vi "FIR_4decimate_Filter2.vi"(8 "valid in":bool, 10 "Q in":fxp<+/-,16,14>, 11 "I in":fxp<+/-,16,14>) -> (0 "valid out":bool, 2 "Q out":fxp<+/-,16,14>, 3 "I out":fxp<+/-,16,14>)   [LabVIEW 2013]
uses:
  <vilib>/rvi/IPIntegrationNode/IPINode_Utilities/niFpgaIPINodeSimCore.vi
  <vilib>/rvi/XilinxIP/XIPIN_XNode/niFpgaXIPIN.xnode
  Filters/Polyphase filterbank/Filter2/Polyphase_filterbank_Filter2_155030D15C70440C8A7262E8A5168E06.dll
  <vilib>/rvi/IPIntegrationNode/IPINode_Xnode/niFpgaIPINode.xnode
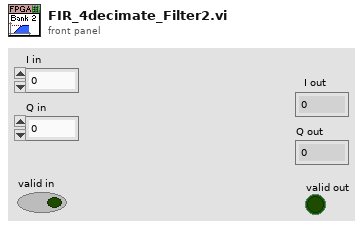
[diagram p1: front panel]
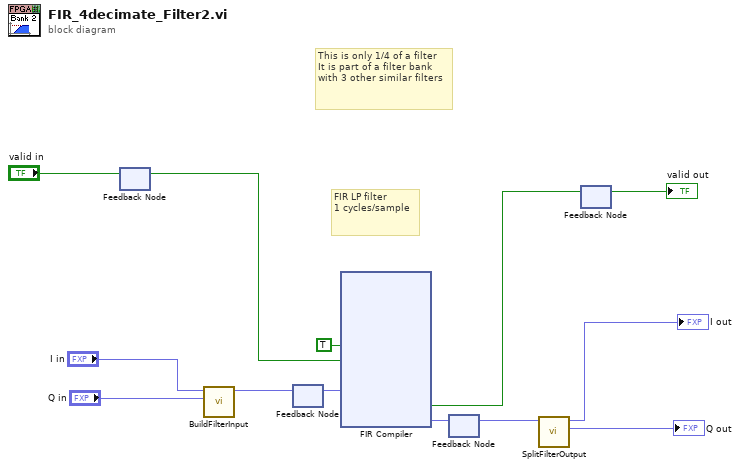
[diagram p0: block diagram]
diagram:
  # "This is only 1/4 of a filter\nIt is part of a filter bank\nwith 3 other similar filters"
  # "FIR LP filter\n1 cycles/sample"
  n1 = feedback-in #1("valid in") -> ()
  n2 = feedback #1() -> (w3:bool)  [unwired: 1 in]
  n3 = call "BuildFilterInput.vi"("Q in"="Q in", "I in"="I in") -> ("Filter input"=w8:fxp<+,32,32>)  [unwired: 9 in]
  n4 = feedback-in #2(w8) -> ()
  n5 = feedback #2() -> (w4:fxp<+,32,32>)  [unwired: 1 in]
  n6 = xnode ("FIR Compiler")("aresetn"=TRUE, "s_axis_data_tvalid"=w3, "s_axis_data_tdata"=w4) -> ("m_axis_data_tvalid"=w7:bool, "m_axis_data_tdata"=w6:fxp<+,64,64>)  [unwired: 1 in, 1 out]
  n7 = feedback-in #3(w6) -> ()
  n8 = feedback #3() -> (w1:fxp<+,64,64>)  [unwired: 1 in]
  n9 = call "SplitFilterOutput.vi"("filter output"=w1) -> ("Q out"=→"Q out":fxp<+/-,16,14>, "I out"=→"I out":fxp<+/-,16,14>)  [unwired: 9 in]
  n10 = feedback-in #4(w7) -> ()
  n11 = feedback #4() -> (→"valid out":bool)  [unwired: 1 in]
